vi "Pasco Auton Drive.vi"(0 "Desired Heading":dbl, 1 "Actual Heading":dbl, 2 "time/distance":dbl, 3 "Power":dbl, 4 "Array":i32, 5 "Encoder":dbl, 7 "Encoder  Returned":dbl) -> (14 "Left Drive":dbl, 15 "Right Drive":dbl, 16 "Array Out":i32, 17 "Encoder total":dbl)   [LabVIEW 2011]
panel:
  in  "Play":dbl
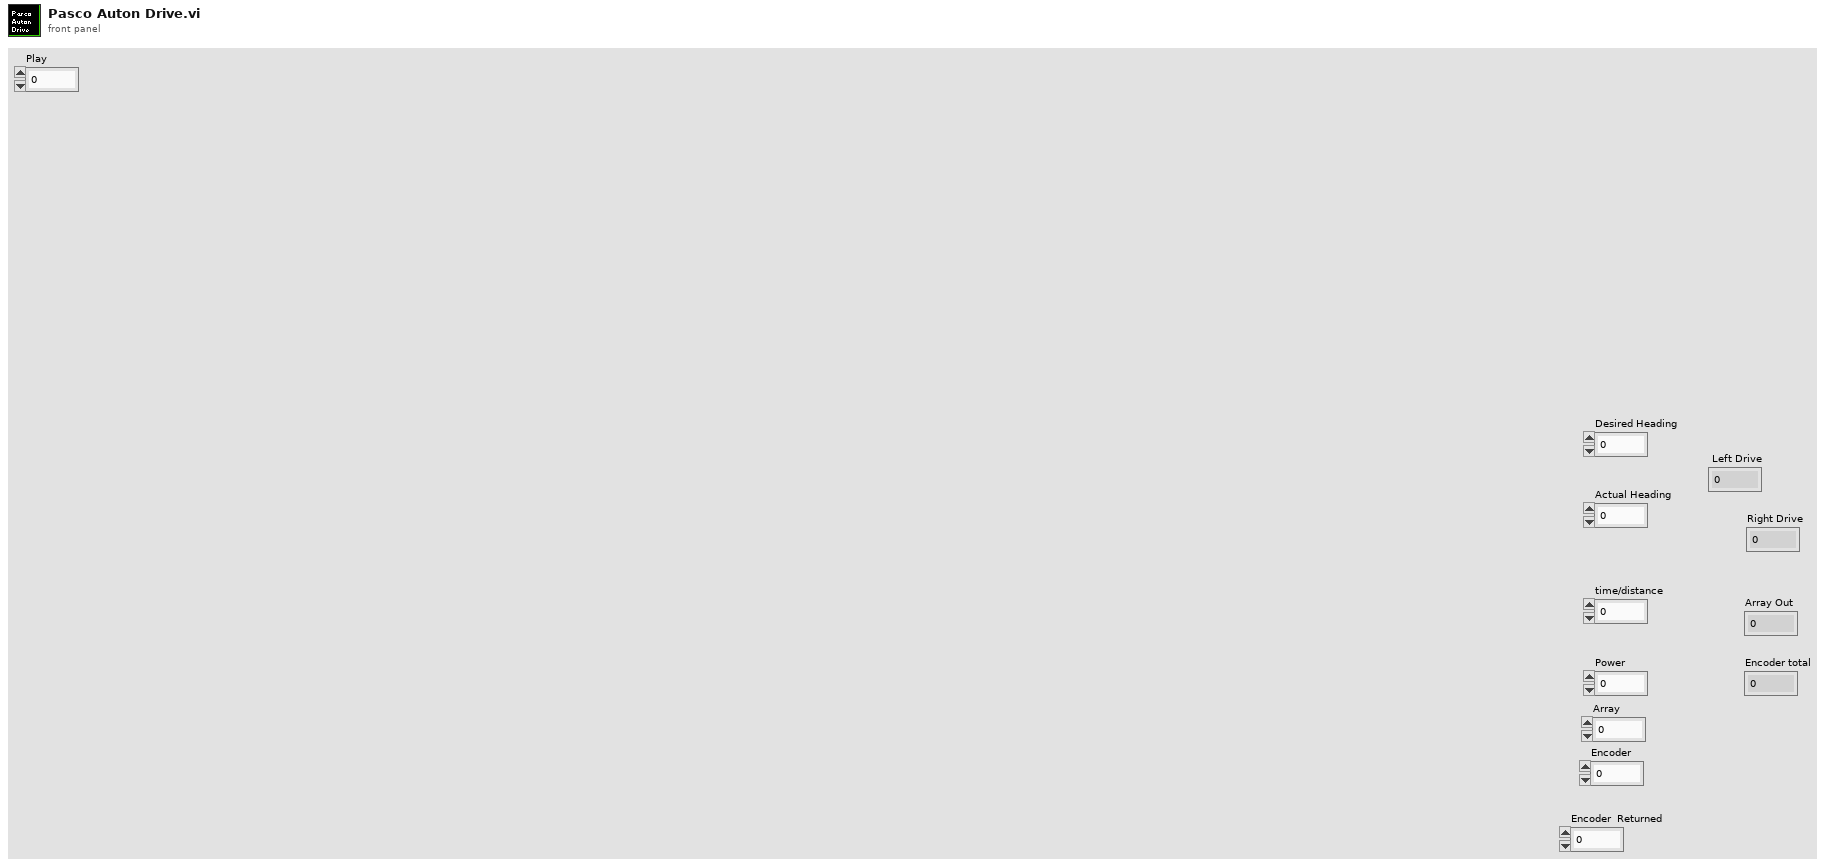
[diagram p1: front panel]
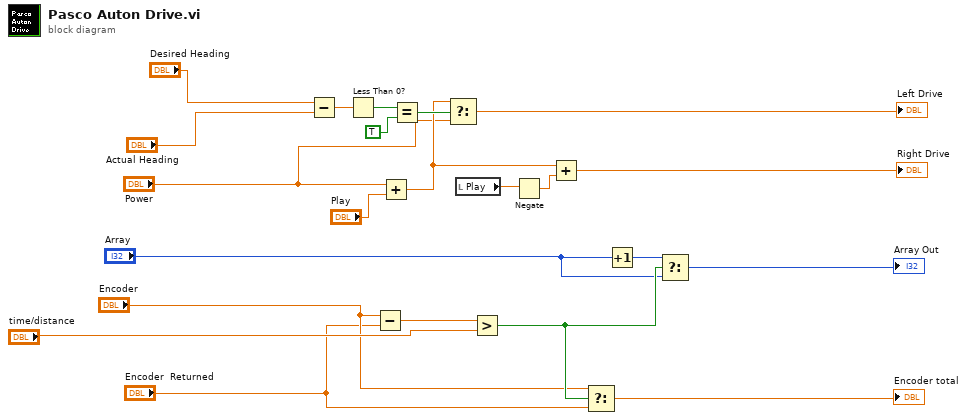
[diagram p0: block diagram]
diagram:
  n1 = Subtract(x="Desired Heading", y="Actual Heading") -> (x-y=w22:dbl)
  n2 = Less Than 0?(x=w22) -> (x < 0?=w21:bool)
  n3 = Subtract(x="Encoder", y="Encoder  Returned") -> (x-y=w14:dbl)
  n4 = Add(x="Power", y="Play") -> (x+y=w16:dbl)
  n5 = Equal?(x=w21, y=TRUE) -> (x = y?=w19:bool)
  n6 = Select(t=w16, s=w19, f="Power") -> (s? t:f=→"Left Drive":dbl)
  n7 = local read "Play"() -> (w15:dbl)
  n8 = Greater?(x=w14, y="time/distance") -> (0:w13:bool)
  n9 = Negate(x=w15) -> (-x=w17:dbl)
  n10 = Add(x=w16, y=w17) -> (x+y=→"Right Drive":dbl)
  n11 = Select(t="Encoder", s=w13, f="Encoder  Returned") -> (s? t:f=→"Encoder total":dbl)
  n12 = Increment(x="Array") -> (x+1=w12:i32)
  n13 = Select(t=w12, s=w13, f="Array") -> (s? t:f=→"Array Out":i32)
